vi "Scan Engine Timing Source.vi"(8 "error in (no error)":errorcluster, 10 "Loop Time (usec)":u32, 11 "Device Ref":T1=18446744073709551615 format="%.0x") -> (0 "error out":errorcluster, 1 "Primary Control Loop dt":i64, 2 "Actual Loop Rate (Hz)":dbl, 3 "Timing Source Name":string, 4 "Do not destroy the custom timing source":bool)   [LabVIEW 2016, in "Scan Engine Custom Device.lvlib"]
uses:
  Scan Engine Custom Device.lvlib
  <vilib>/NI Veristand/Custom Device API/Custom Device Item Ref.ctl
  Globals/RT Globals.vi
  <vilib>/NI Veristand/Custom Device API/Custom Device API.lvlib
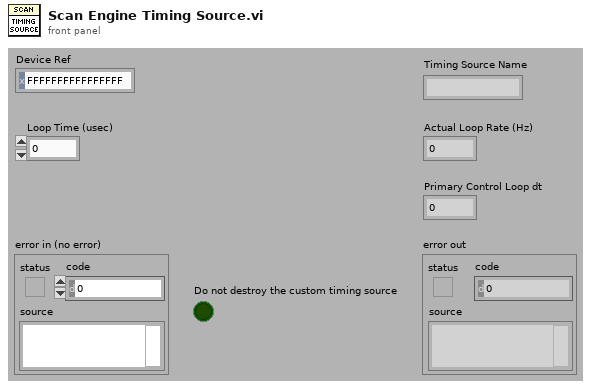
[diagram p1: front panel]
types:
  T1 = typedef "Custom Device API.lvlib/Custom Device Item Ref.ctl" = u64
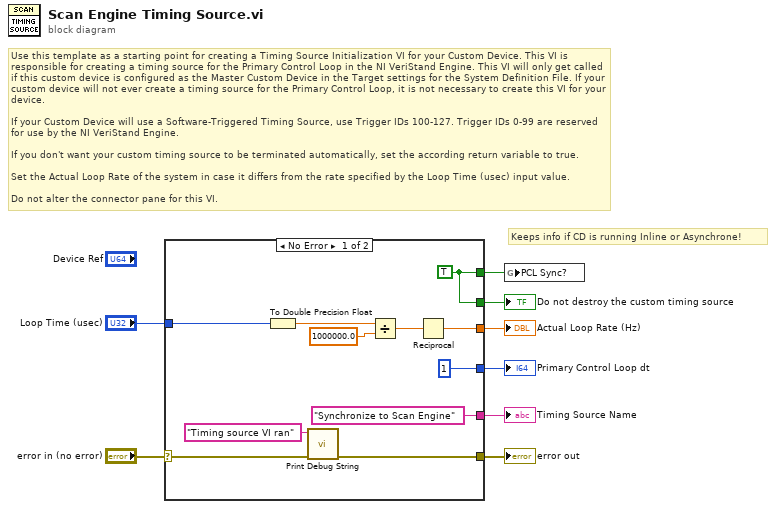
[diagram p0: block diagram]
diagram:
  # "Keeps info if CD is running Inline or Asynchrone!"
  # "Use this template as a starting point for creating a Timing Source Initialization VI for your Custom Device. This VI is responsible for creating a timing source for the Primary Control Loop in the NI VeriStand Engine. This VI will only get called if this custom device is configured as the Master Custom Device in the Target settings for the System Definition File. If your custom device will not ever create a timing source for the Primary Control Loop, it is not necessary to create this VI for your device.\n\nIf your Custom Device will use a Software-Triggered Timing Source, use Trigger IDs 100-127. Trigger IDs 0-99 are reserved for use by the NI VeriStand Engine.\n\nIf you don't want your custom timing source to be terminated automatically, set the according return variable to true.\n\nSet the Actual Loop Rate of the system in case it differs from the rate specified by the Loop Time (usec) input value.\n\nDo not alter the connector pane for this VI."
  n1 = case shown="No Error" "error in (no error)" {
    selector: "error in (no error)" -> [w9 w20]
    tunnel: [w14 w20] -> w8
    tunnel: "Loop Time (usec)" -> [w15 _]
    tunnel: [w13 _] -> w5
    tunnel: ["Synchronize to Scan Engine" ("Source Name") _] -> w4
    tunnel: [i64 1 ("Primary Control Loop dt") _] -> w3
    tunnel: [w11 _] -> w2
    tunnel: [w11 _] -> w1
    frame No Error {
      w11 = TRUE ("PCL Sync?")
      n2 = To Double Precision Float(number=w15) -> (double precision float=w16:dbl)
      n3 = call "Print Debug String.vi"("error in"=w9, "String to write"="Timing source VI ran") -> ("error out"=w14:errorcluster)  [unwired: 8 in]
      n4 = Divide(x=w16, y=1000000.0) -> (x/y=w18:dbl)
      n5 = Reciprocal(x=w18) -> (1/x=w13:dbl)
    }
    frame Error {
    }
  }
  "error out" <- w8
  "Timing Source Name" <- w4
  "Actual Loop Rate (Hz)" <- w5
  "Primary Control Loop dt" <- w3
  "Do not destroy the custom timing source" <- w1
  n6 = global write "RT Globals.vi" "PCL Sync?"(w2) -> ()
